vi "_Connect_DB.vi"(8 "error in (no error)":errorcluster, 11 "Postgres Connector In":refnum<class "Postgres Connector.lvclass">) -> (0 "error out":errorcluster, 3 "Postgres Connector Out":refnum<class "Postgres Connector.lvclass">)   [LabVIEW 2019, in "PG_LIB.lvlib" / "Postgres Connector.lvclass"]
doc: "This VI build the string so the user can connect to the database."
uses:
  Postgres Connector.lvclass
  Postgres Connector.lvclass/Postgres Connector.ctl
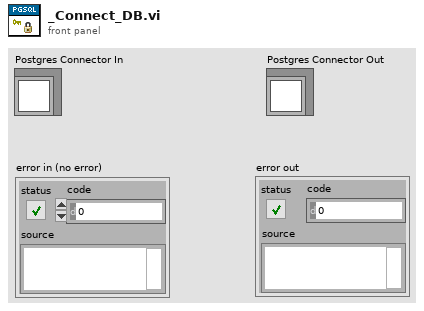
[diagram p1: front panel]
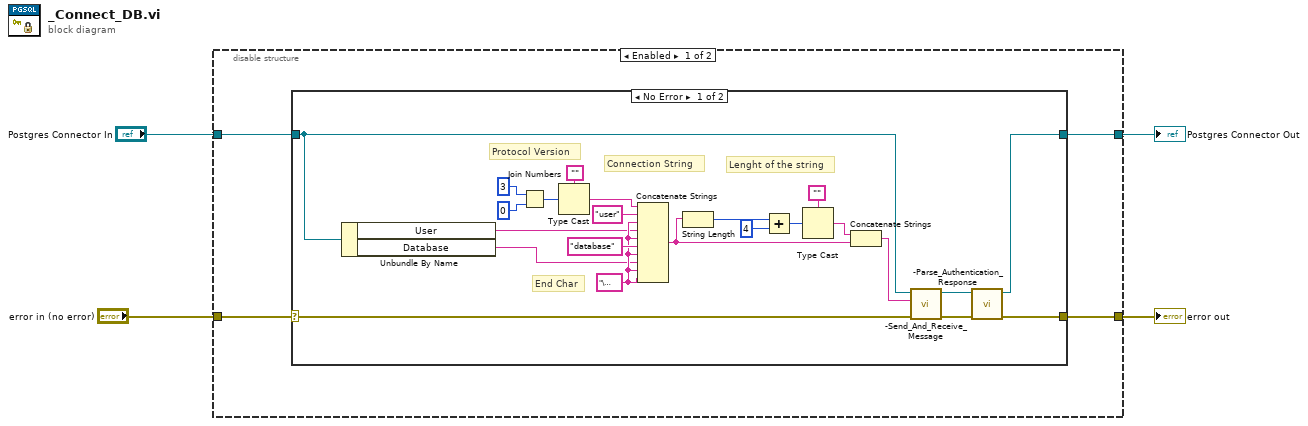
[diagram p0: block diagram]
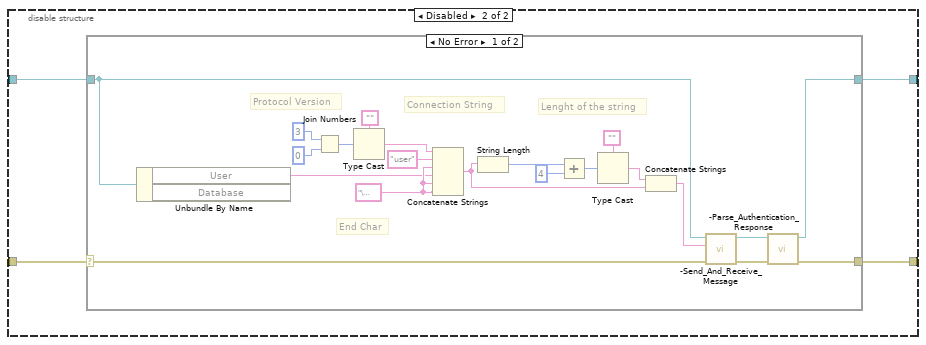
[diagram p3: hidden frame]
diagram:
  n1 = disable-structure shown="Enabled" {
    disable-tunnel: "error in (no error)" -> [w8 w37]
    disable-tunnel: [w7 w36] -> w3
    disable-tunnel: "Postgres Connector In" -> [w6 w35]
    disable-tunnel: [w5 w34] -> w1
    frame Enabled {
      n2 = case shown="No Error" w8 {
        selector: w8 -> [w15 w32]
        tunnel: [w12 w32] -> w7
        tunnel: w6 -> [w14 w33]
        tunnel: [w9 w33] -> w5
        frame No Error {
          w18 = "\u0000"
          # "Lenght of the string"
          # "Connection String"
          # "Protocol Version"
          # "End Char"
          n3 = Unbundle By Name(w14) -> ("User"=w17:string, "Database"=w16:string)
          n4 = Join Numbers(hi=i16 3, lo=i16 0) -> ((hi.lo)=w27:u32)
          n5 = Type Cast(type="", x=w27) -> (*(type *) &x=w25:string)
          n6 = Concatenate Strings(w25, "user", w18, w17, w18, "database", w18, w16, w18, w18) -> (w22:string)
          n7 = String Length(string=w22) -> (length=w21:i32)
          n8 = Add(x=w21, y=4) -> (x+y=w19:i32)
          n9 = Type Cast(type="", x=w19) -> (*(type *) &x=w23:string)
          n10 = Concatenate Strings(w23, w22) -> (w13:string)
          n11 = call "-Send_And_Receive_Message.vi"("error in (no error)"=w15, "Message To Send"=w13, "Postgres Connector In"=w14) -> ("error out"=w11:errorcluster, "Postgres Connector Out"=w10:refnum<class "Postgres Connector.lvclass">)  [unwired: 6 in, 1 out]
          n12 = call "-Parse_Authentication_Response.vi"("error in (no error)"=w11, "Postgres Connector In"=w10) -> ("error out"=w12:errorcluster, "Postgres Connector Out"=w9:refnum<class "Postgres Connector.lvclass">)  [unwired: 8 in]
        }
        frame Error {
        }
      }
    }
    frame Disabled {
      n13 = case shown="No Error" w37 {
        selector: w37 -> [w44 w59]
        tunnel: [w41 w59] -> w36
        tunnel: w35 -> [w43 w60]
        tunnel: [w38 w60] -> w34
        frame No Error {
          w46 = "\u0000"
          # "Lenght of the string"
          # "Connection String"
          # "Protocol Version"
          # "End Char"
          n14 = Unbundle By Name(w43) -> ("User"=w45:string)  [unwired: 1 out]
          n15 = Join Numbers(hi=i16 3, lo=i16 0) -> ((hi.lo)=w55:u32)
          n16 = Type Cast(type="", x=w55) -> (*(type *) &x=w53:string)
          n17 = Concatenate Strings(w53, "user", w46, w45, w46, w46) -> (w50:string)
          n18 = String Length(string=w50) -> (length=w49:i32)
          n19 = Add(x=w49, y=4) -> (x+y=w47:i32)
          n20 = Type Cast(type="", x=w47) -> (*(type *) &x=w51:string)
          n21 = Concatenate Strings(w51, w50) -> (w42:string)
          n22 = call "-Send_And_Receive_Message.vi"("error in (no error)"=w44, "Message To Send"=w42, "Postgres Connector In"=w43) -> ("error out"=w40:errorcluster, "Postgres Connector Out"=w39:refnum<class "Postgres Connector.lvclass">)  [unwired: 6 in, 1 out]
          n23 = call "-Parse_Authentication_Response.vi"("error in (no error)"=w40, "Postgres Connector In"=w39) -> ("error out"=w41:errorcluster, "Postgres Connector Out"=w38:refnum<class "Postgres Connector.lvclass">)  [unwired: 8 in]
        }
        frame Error {
        }
      }
    }
  }
  "error out" <- w3
  "Postgres Connector Out" <- w1
